vi "NotFound.vi"() -> ()   [LabVIEW 2019]
panel:
  in  "OK Button":bool
  # "Nie znaleziono takiego \n           produktu"
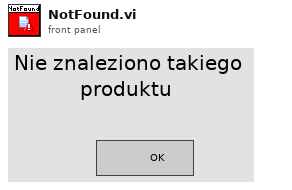
[diagram p1: front panel]
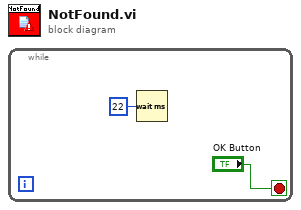
[diagram p0: block diagram]
diagram:
  n1 = while {
    stop <- "OK Button" stop-if-true
    n2 = Wait (ms)(milliseconds to wait=u32 22) -> ()  [unwired: 1 out]
  }
